vi "Post Message To Slack.vi"(11 "error in (no error)":errorcluster) -> (15 "error out":errorcluster)   [LabVIEW 2013]
uses:
  <vilib>/httpClient/ClientHandle.ctl
  postMessageCluster.ctl
  <vilib>/Utility/config.llb/Read Key (String).vi
  <vilib>/Utility/config.llb/Read Key (Boolean).vi
  <vilib>/httpClient/POSTBuffer.vi
  <vilib>/httpClient/LabVIEWHTTPClient.lvlib
  <vilib>/Utility/config.llb/NI_LVConfig.lvlib
panel:
  out "client handle out":T1
  out "headers":string
  out "body":string
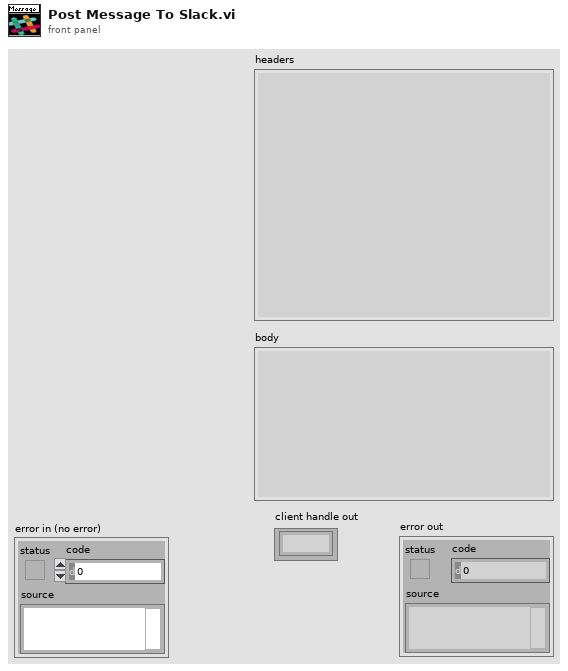
[diagram p1: front panel]
types:
  T1 = typedef "LabVIEWHTTPClient.lvlib/ClientHandle.ctl" = refnum<k1>
  T2 = typedef "postMessageCluster.ctl" = cluster{"token":string, "channel":string, "text":string, "as_user":bool, "username":string}
  T3 = typedef "NI_LVConfig.lvlib/Config Data RefNum.ctl" = refnum<k1>
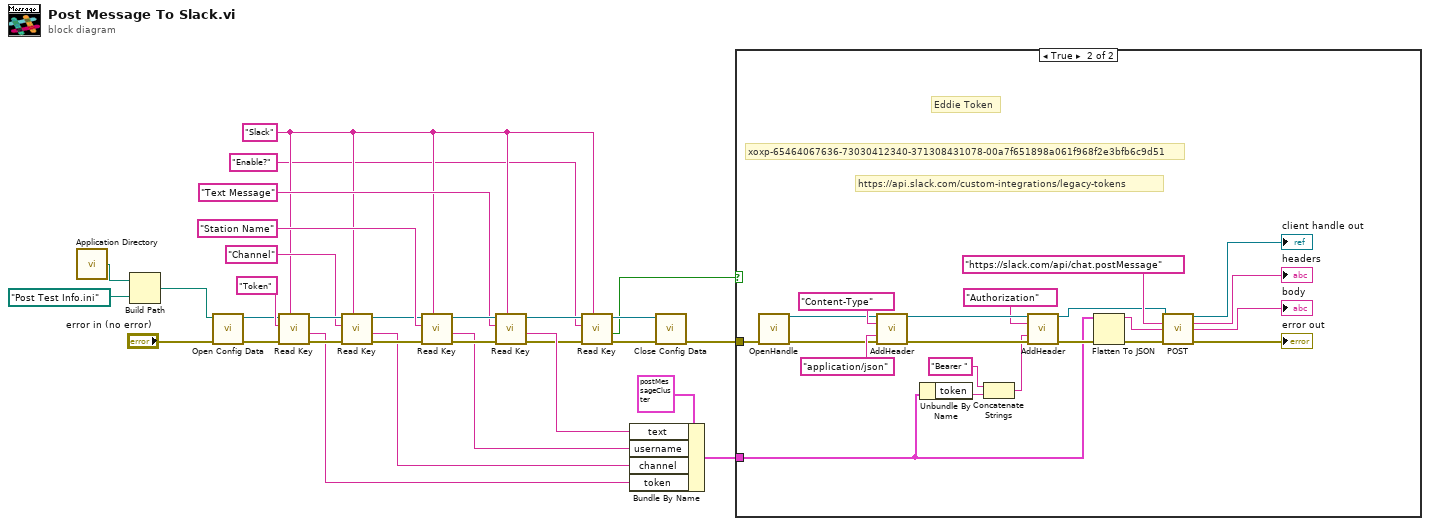
[diagram p0: block diagram]
diagram:
  w3 = "Slack" ("section")
  n1 = call <vilib>:"Application Directory.vi"() -> ("Application Directory"=w10:path)
  n2 = Build Path(base path=w10, name or relative path=path "Post Test Info.ini" ("default name")) -> (appended path=w9:path)
  n3 = call <vilib>:"Open Config Data.vi"("error in (no error)"="error in (no error)", "configuration file path"=w9) -> ("error out"=w25:errorcluster, "refnum"=w26:T3)  [unwired: 7 in, 1 out]
  n4 = call-poly <vilib>:"Read Key.vi"("section"=w3, "error in (no error)"=w25, "key"="Token", "refnum"=w26) -> ("error out"=w29:errorcluster, "value"=w12:string, "refnum out"=w28:T3)  [unwired: 4 in, 1 out]
  n5 = call-poly <vilib>:"Read Key.vi"("section"=w3, "error in (no error)"=w29, "key"="Channel", "refnum"=w28) -> ("error out"=w20:errorcluster, "value"=w13:string, "refnum out"=w19:T3)  [unwired: 4 in, 1 out]
  n6 = call-poly <vilib>:"Read Key.vi"("section"=w3, "error in (no error)"=w20, "key"="Station Name", "refnum"=w19) -> ("error out"=w18:errorcluster, "value"=w14:string, "refnum out"=w17:T3)  [unwired: 4 in, 1 out]
  n7 = call-poly <vilib>:"Read Key.vi"("section"=w3, "error in (no error)"=w18, "key"="Text Message", "refnum"=w17) -> ("error out"=w6:errorcluster, "value"=w15:string, "refnum out"=w5:T3)  [unwired: 4 in, 1 out]
  n8 = call-poly <vilib>:"Read Key.vi"("section"=w3, "error in (no error)"=w6, "key"="Enable?", "refnum"=w5) -> ("error out"=w7:errorcluster, "value"=w2:bool, "refnum out"=w4:T3)  [unwired: 4 in, 1 out]
  n9 = Bundle By Name(cluster=T2 {"token"="xoxp-65464067636-73030412340-371308431078-00a7f651898a061f968f2e3bfb6c9d51", "channel"="dallas_lab", "text"="This message is posted by LabView", "as_user"=FALSE, "username"="Dinesh"} ("postMessageCluster"), "text"=w15, "username"=w14, "channel"=w13, "token"=w12) -> (w21:T2)
  n10 = call <vilib>:"Close Config Data.vi"("error in (no error)"=w7, "refnum"=w4) -> ("error out"=w23:errorcluster)  [unwired: 8 in, 1 out]
  n11 = case shown="True" w2 {
    tunnel: w23 -> [_ w32]
    tunnel: w21 -> [_ w31]
    frame False {
    }
    frame True {
      # "https://api.slack.com/custom-integrations/legacy-tokens"
      # "Eddie Token"
      # "xoxp-65464067636-73030412340-371308431078-00a7f651898a061f968f2e3bfb6c9d51"
      n12 = call <vilib>:"OpenHandle.vi"("error in (no error)"=w32) -> ("client handle out"=w42:T1, "error out"=w38:errorcluster)  [unwired: 13 in]
      n13 = call <vilib>:"AddHeader.vi"("client handle"=w42, "header"="Content-Type", "value"="application/json", "error in (no error)"=w38) -> ("client handle out"=w40:T1, "error out"=w39:errorcluster)  [unwired: 10 in]
      n14 = Unbundle By Name(w31) -> ("token"=w34:string)
      n15 = Concatenate Strings("Bearer " ("string"), w34) -> (w36:string)
      n16 = call <vilib>:"AddHeader.vi"("client handle"=w40, "header"="Authorization", "value"=w36, "error in (no error)"=w39) -> ("client handle out"=w41:T1, "error out"=w33:errorcluster)  [unwired: 10 in]
      n17 = Flatten To JSON(anything=w31, error in (no error)=w33) -> (JSON string=w46:string, 11:w45:errorcluster)  [unwired: 1 in]
      n18 = call-poly <vilib>:"POST.vi"("client handle"=w41, "url"="https://slack.com/api/chat.postMessage", "buffer"=w46, "error in (no error)"=w45) -> ("client handle out"=→"client handle out":T1, "headers"=→"headers":string, "body"=→"body":string, "error out"=→"error out":errorcluster)  [unwired: 8 in]
    }
  }
